vi "RSSI.vi"(8 "error in":errorcluster) -> (0 "error out":errorcluster, 2 "link":dbl)   [LabVIEW 2017]
doc: "Use this VI to retrieve wireless quality information on myRIO devices with WiFi.\nThe information is based on: cat /proc/net/wireless"
panel:
  in  "?":bool
  out "dBM":dbl
  out "Gauge":dbl(knob) scale=-10.0..-90.0
  # "Good"
  # "Weak"
  # "Excellent"
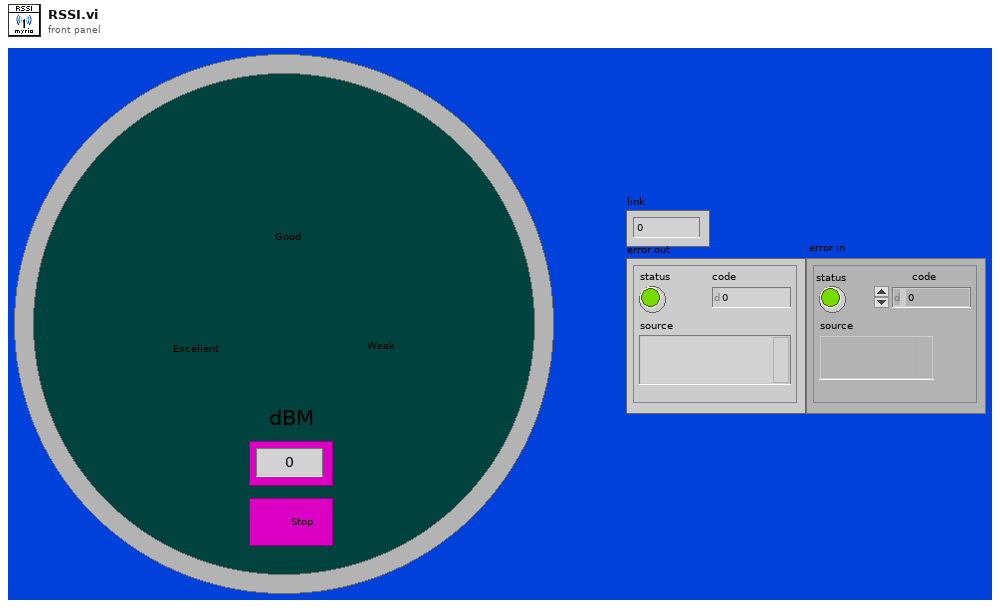
[diagram p1: front panel]
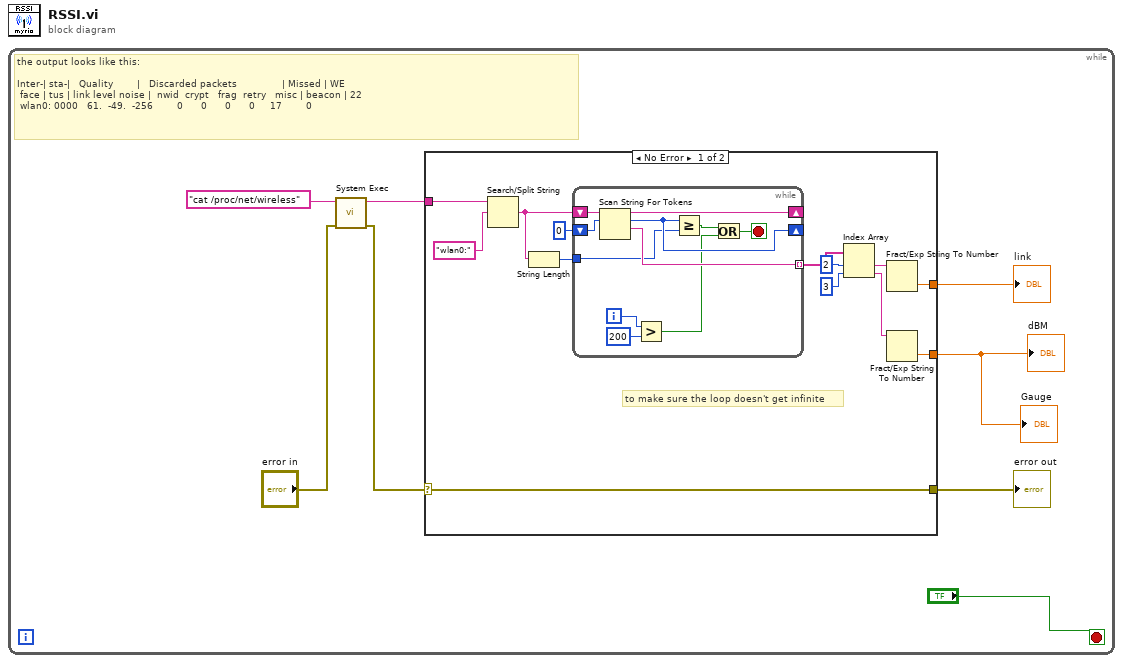
[diagram p0: block diagram]
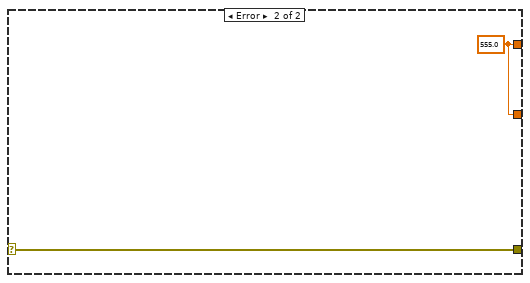
[diagram p2: hidden frame]
diagram:
  n1 = while {
    stop <- "?" stop-if-true
    # "the output looks like this:\n\nInter-| sta-|   Quality        |   Discarded packets               | Missed | WE\n face | tus | link level noise |  nwid  crypt   frag  retry   misc | beacon | 22\n wlan0: 0000   61.  -49.  -256        0      0      0      0     17        0"
    n2 = call <vilib>:"System Exec.vi"("error in (no error)"="error in", "command line"="cat /proc/net/wireless") -> ("error out"=w5:errorcluster, "standard output"=w7:string)  [unwired: 6 in, 2 out]
    n3 = case shown="No Error" w5 {
      selector: w5 -> [w9 w33]
      tunnel: w7 -> [w21 _]
      tunnel: [w12 w34] -> w6
      tunnel: [w11 w34] -> w1
      tunnel: [w9 w33] -> w4
      frame No Error {
        # "to make sure the loop doesn't get infinite"
        n4 = Search/Split String(string=w21, search string/char (-)="wlan0:" ("search string")) -> (match + rest of string=w18:string)  [unwired: 1 in, 2 out]
        n5 = String Length(string=w18) -> (length=w17:i32)
        n6 = while {
          shift-right: [w31] -> _
          shift-left: w18 -> [w32]
          tunnel: [w30] -> w16 mode=indexing
          shift-right: [w28] -> _
          shift-left: 0 ("offset past token") -> [w29]
          tunnel: w17 -> [w27]
          i -> [w25]
          stop <- w23 stop-if-true
          n7 = Scan String For Tokens(8:w29, 9:w32) -> (1:w30:string, 2:w28:i32, 3:w31:string)  [unwired: 4 in, 1 out]
          n8 = Greater?(x=w25, y=200) -> (0:w22:bool)
          n9 = Greater Or Equal?(x=w28, y=w27) -> (x >= y?=w26:bool)
          n10 = Or(x=w26, y=w22) -> (x .or. y?=w23:bool)
        }
        n11 = Index Array(array=w16, index #1=2 ("index"), index #2=3 ("index")) -> (element #1=w13:string, element #2=w10:string)
        n12 = Fract/Exp String To Number(string=w13) -> (number=w12:dbl)  [unwired: 3 in, 1 out]
        n13 = Fract/Exp String To Number(string=w10) -> (number=w11:dbl)  [unwired: 3 in, 1 out]
      }
      frame Error {
        w34 = 555.0
      }
    }
    "link" <- w6
    "error out" <- w4
    "Gauge" <- w1
    "dBM" <- w1
  }
